vi "Job Initialize UI.vi"() -> ()   [LabVIEW 2014, in "Job Initialize.lvclass"]
uses:
  Job Initialize.lvclass
  <vilib>/ni/Configuration Framework/Node/NodeRef.ctl
  <vilib>/ni/Configuration Framework/Node/NISE_CEF_Node.lvclass
  <vilib>/ni/AMC/Message Queue.ctl
  <vilib>/ni/AMC/Message.ctl
  <vilib>/ni/Tools/Keyed Array/KeyedArray.ctl
  <vilib>/ni/Configuration Framework/Node/UserEventRef.ctl
  <vilib>/ni/Configuration Framework/Controls/EventCluster.ctl
  Controls/Cron String - STYP.ctl
  Controls/Source Code Control Selection - STYP.ctl
  Job Initialize.lvclass/Job Initialize.ctl
  Build Job/Build Job.lvclass/Build Job.ctl
  Build Job/Build Job.lvclass
  <vilib>/ni/Tools/Keyed Array/Tools_KeyedArray.lvlib
  <vilib>/ni/AMC/AMC.lvlib
  <vilib>/ni/Configuration Framework/NISE_CEF_TreeControl.lvlib
panel:
  in  "Description":string="brandyn.adderley@ni.com"
  in  "Source Code Poll":T1
  in  "Build Trigger":T2={"Day of Week"=enum."Everyday", "Hour"=23, "Enable?"=FALSE} {"Hour" min=0 max=23}
  in  "user event":T3
  in  "main queue":T4
  in  "node ref":T5
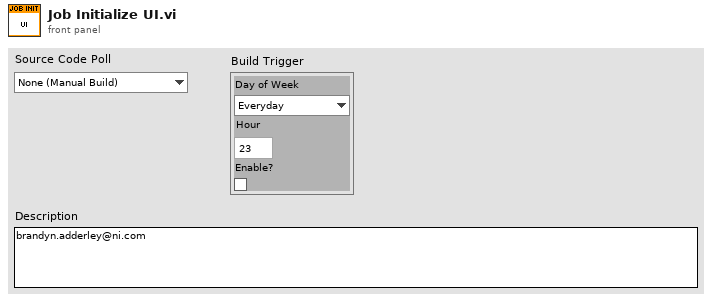
[diagram p1: front panel]
types:
  T1 = typedef "Source Code Control Selection - STYP.ctl" = enum16{"None (Manual Build)", "Every 15 Minutes", "Every 30 Minutes", "Every 45 Minutes", "Every Hour", "Every 2 Hours", "Everyday "}
  T2 = typedef "Cron String - STYP.ctl" = cluster{"Day of Week":enum16{"Everyday", "Sunday", "Monday", "Tuesday", "Wednesday", "Thursday", "Friday", "Saturday"}, "Hour":i32, "Enable?":bool}
  T3 = typedef "NISE_CEF_Node.lvclass/UserEventRef.ctl" = refnum<user-event>
  T4 = typedef "AMC.lvlib/Message Queue.ctl" = refnum<queue>
  T5 = typedef "NISE_CEF_Node.lvclass/NodeRef.ctl" = refnum<data-value>
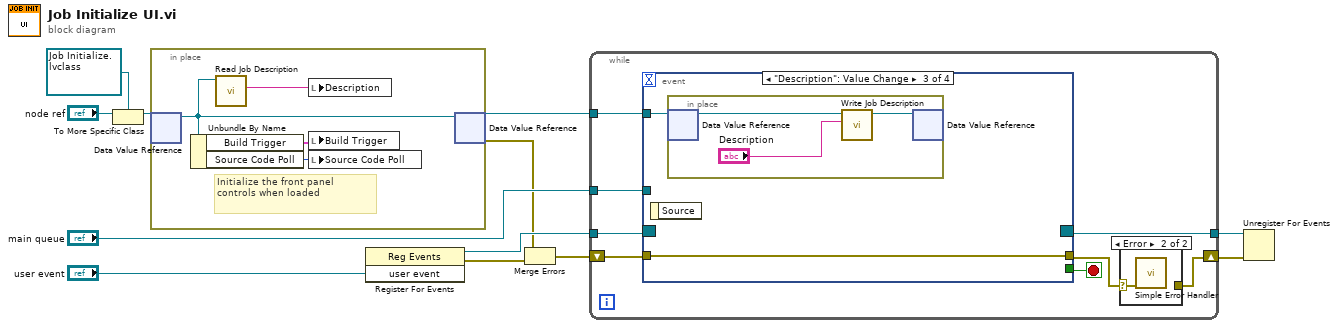
[diagram p0: block diagram]
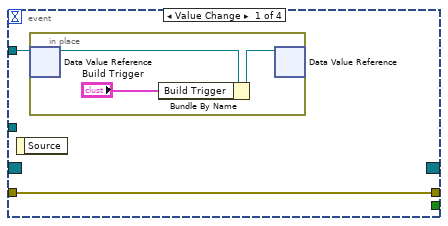
[diagram p3: hidden frame]
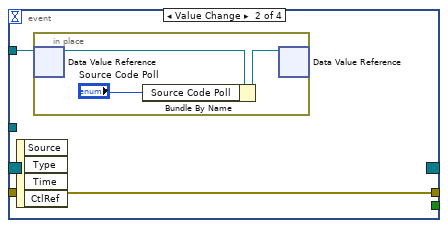
[diagram p4: hidden frame]
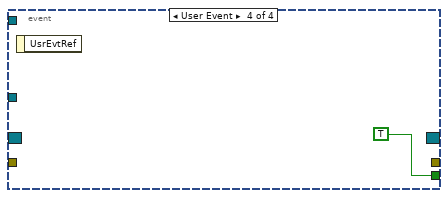
[diagram p5: hidden frame]
diagram:
  n1 = To More Specific Class(target class=refnum<data-value> refnum ("data value reference"), reference="node ref") -> (specific class reference=w5:refnum<data-value>)  [unwired: 1 in, 1 out]
  n2 = in-place {
    # "Initialize the front panel controls when loaded"
    n3 = in-place-dvr #1(w5) -> (w14:refnum<class "Job Initialize.lvclass">)  [unwired: 1 out]
    n4 = Unbundle By Name(w14) -> ("Build Trigger"=w16:T2, "Source Code Poll"=w15:T1)
    n5 = call-dynamic "Read Job Description.vi"("Build Job in"=w14) -> ("Job Description"=w13:string)  [unwired: 10 in]
    n6 = local write "Description"(w13) -> ()
    n7 = local write "Build Trigger"(w16) -> ()
    n8 = local write "Source Code Poll"(w15) -> ()
    n9 = in-place-dvr #1(w14) -> (w12:refnum<data-value>, w2:errorcluster)
  }
  n10 = register-events("user event") -> (reference out=w9:refnum<event-registration>, error out=w3:errorcluster)  [unwired: 2 in]
  n11 = Merge Errors(w2, w3) -> (w1:errorcluster)
  n12 = while {
    tunnel: w12 -> [w24]
    tunnel: "main queue" -> [w23]
    tunnel: w9 -> [w22]
    tunnel: [w21] -> w8
    shift-right: [w17] -> w7
    shift-left: w1 -> [w20]
    stop <- w19 stop-if-true
    n13 = event shown="[2] \"Description\": Value Change" {
      selector: w22 -> [_ _ _ _]
      dyn-events: [_ _ _ _] -> w21
      timeout: _ -> [_ _ _ _]
      tunnel: w24 -> [w28 w33 w38 _]
      tunnel: w23 -> [_ _ _ _]
      tunnel: [_ _ _ TRUE] -> w19
      tunnel: [w27 w32 w37 _] -> w18
      tunnel: w20 -> [w27 w32 w37 _]
      event Value Change {
        n14 = event-data() -> ()  [unwired: 1 in, 1 out]
        n15 = in-place {
          n16 = in-place-dvr #2(w28) -> (w31:refnum<class "Job Initialize.lvclass">)  [unwired: 1 out]
          n17 = Bundle By Name(cluster=w31, "Build Trigger"="Build Trigger") -> (w30:refnum<class "Job Initialize.lvclass">)
          n18 = in-place-dvr #2(w30) -> ()  [unwired: 2 out]
        }
      }
      event Value Change {
        n19 = event-data() -> ()  [unwired: 1 in, 4 out]
        n20 = in-place {
          n21 = in-place-dvr #3(w33) -> (w36:refnum<class "Job Initialize.lvclass">)  [unwired: 1 out]
          n22 = Bundle By Name(cluster=w36, "Source Code Poll"="Source Code Poll") -> (w35:refnum<class "Job Initialize.lvclass">)
          n23 = in-place-dvr #3(w35) -> ()  [unwired: 2 out]
        }
      }
      event "Description": Value Change {
        n24 = event-data() -> ()  [unwired: 1 in, 1 out]
        n25 = in-place {
          n26 = in-place-dvr #4(w38) -> (w41:refnum<class "Job Initialize.lvclass">)  [unwired: 1 out]
          n27 = call "Write Job Description.vi"("Job Description"="Description", "Build Job in"=w41) -> ("Build Job out"=w40:refnum<class "Job Initialize.lvclass">)  [unwired: 9 in]
          n28 = in-place-dvr #4(w40) -> ()  [unwired: 2 out]
        }
      }
      event User Event {
        n29 = event-data() -> ()  [unwired: 1 in, 1 out]
      }
    }
    n30 = case shown="Error" w18 {
      selector: w18 -> [w25 w26]
      tunnel: [w25 _] -> w17
      frame No Error {
      }
      frame Error {
        n31 = call <vilib>:"Simple Error Handler.vi"("error in (no error)"=w26) -> ()  [unwired: 4 in, 5 out]
      }
    }
  }
  n32 = Unregister For Events(event registration refnum=w8, error in=w7) -> ()  [unwired: 1 out]
